vi "StoreData_Local.vi"(6 "error in (no error)":errorcluster, 8 "Fname Increment":u8, 9 "Array":dbl[][](array[numeric]), 10 "Save Type":u16(ring)=1 items=["USB", "cRIO"], 11 "Filename":string) -> (0 "NewFnameCount":u8, 1 "New Fname":string, 2 "New Save Type":u16, 3 "Current Free Space (Mb)":dbl, 4 "error out":errorcluster, 5 "Low on Free Disk Space":bool)   [LabVIEW 2013]
uses:
  <vilib>/Utility/file.llb/Write To Spreadsheet File (DBL).vi
panel:
  in  "Bin Header":i32=2
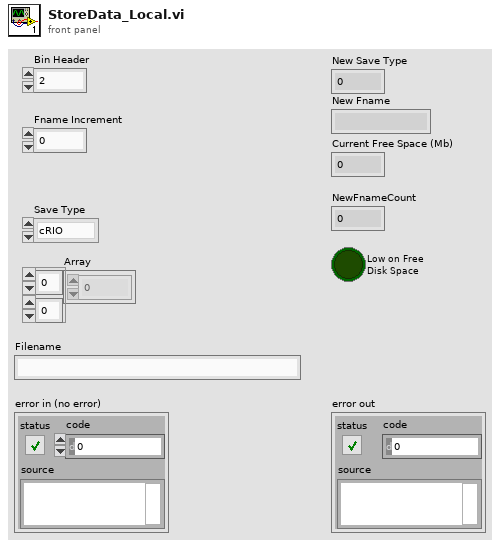
[diagram p1: front panel]
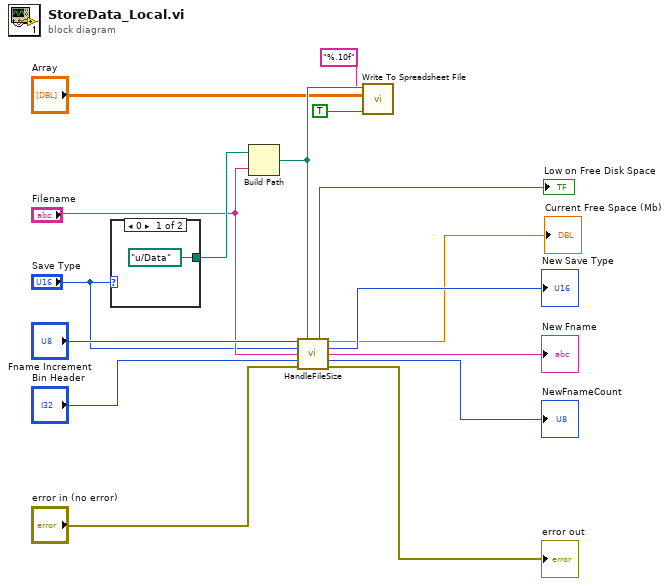
[diagram p0: block diagram]
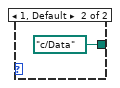
[diagram p2: hidden frame]
diagram:
  n1 = case shown="0" "Save Type" {
    tunnel: [path "u:/Data" path "c:/Data"] -> w12
    frame 0 {
    }
    frame 1, Default {
    }
  }
  n2 = Build Path(base path=w12, name or relative path="Filename") -> (appended path=w14:path)
  n3 = call "HandleFileSize.vi"("FName Increment Count"="Fname Increment", "path"=w14, "Save Type"="Save Type", "Filename"="Filename", "Bin Header"="Bin Header", "error in"="error in (no error)") -> ("Low on Free Disk Space"=→"Low on Free Disk Space":bool, "Current Free Space (Mb)"=→"Current Free Space (Mb)":dbl, "New Save Type"=→"New Save Type":u16, "New Fname"=→"New Fname":string, "NewFnameCount"=→"NewFnameCount":u8, "error out"=→"error out":errorcluster)  [unwired: 4 in]
  n4 = call-poly <vilib>:"Write To Spreadsheet File.vi"("format (%.3f)"="%.10f", "append to file? (new file:F)"=TRUE, "2D data"="Array", "file path (dialog if empty)"=w14) -> ()  [unwired: 4 in, 1 out]
